vi "helper-unit-dose.vi"(6 "Auto Update Limit Record? (T)":bool=TRUE, 8 "error in":errorcluster, 9 "output":string, 10 "Unit Index":i32, 11 "Proc Name":string) -> (0 "error out":errorcluster, 1 "resulting string":string, 2 "Actual Dose in Seconds":i32)   [LabVIEW 2024]
uses:
  controls/enum-ntr-io-format.ctl
  globals/globals-engine.vi
panel:
  out "dose counter":dbl
  out "Daily Limit":dbl
  out "required dose":dbl
  out "ShouldDose":bool
  # "using unitIndex and output arguments this vi will check the daily limit to calculate the dose.\nreturn 0:  if limit is reached (meaning zero dose is no dose)\nretun X: where (0 < X <= doseTime) if limit isn't reached for today\nand keep a log of the process"
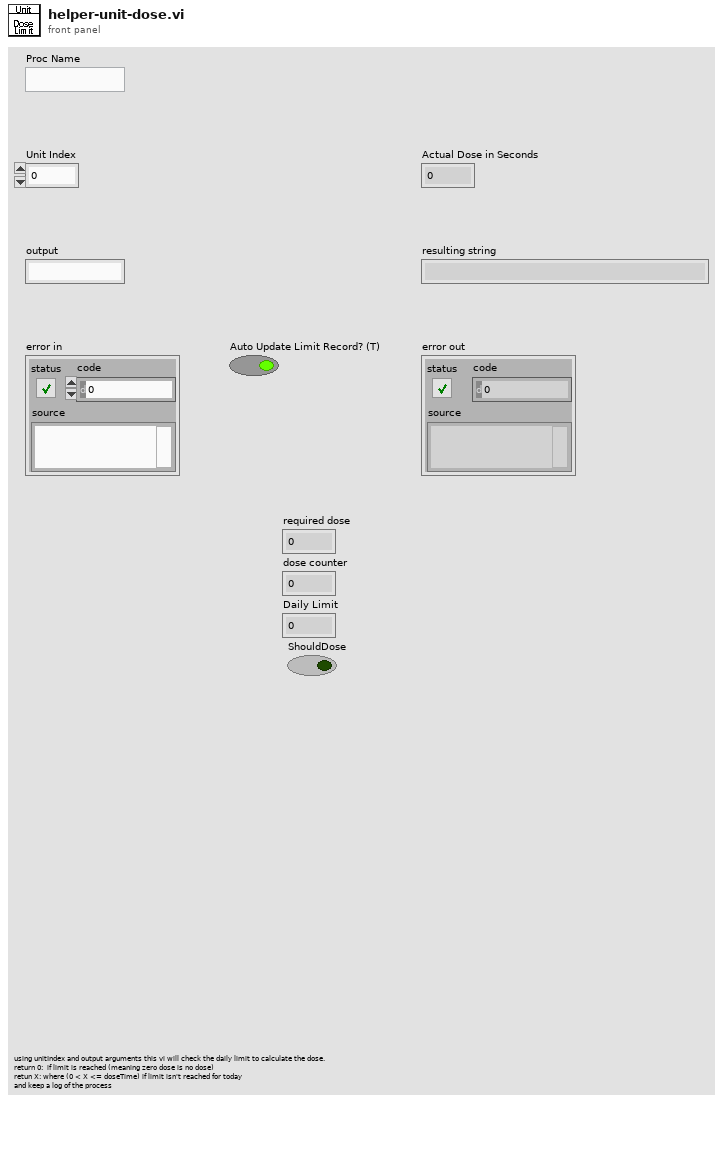
[diagram p1: front panel]
types:
  T1 = typedef "enum-ntr-io-format.ctl" = enum16{"UN_VLV%d", "UN_PMP%d", "UN_WL%d", "UN_PH", "UN_EC", "UN_ORP", "UN_WT", "UN_PH2", "UN_ALFA1", "UN_BETA1", "UN_ALFA2", "UN_BETA2", "UN_ACID", "UN_BASE", "UN_WATER", "UN_ORPMIX"}
  T2 = typedef "UiNutritionPanel.ctl" = cluster{"Main":cluster{"Enable":bool, "WashTimes":cluster{"In":dbl, "Out":dbl}, "DailyActivityHours":cluster{"Begin Time":T3, "End Time":T3}[]}, "Water Dosing":cluster{"Water Dose":dbl, "Water Limit":dbl}, "EC Ranges":cluster{"H Alarm":dbl, "L Alarm":dbl, "Low":dbl}, "EC Dosing":cluster{"ALFA1 Dose":dbl, "ALFA1 Limit":dbl, "BETA1 Dose":dbl, "BETA1 Limit":dbl, "ALFA2 Dose":dbl, "ALFA2 Limit":dbl, "BETA2 Dose":dbl, "BETA2 Limit":dbl}, "PH Ranges":cluster{"H Alarm":dbl, "L Alarm":dbl, "High":dbl, "Low":dbl}, "PH Dosing":cluster{"ACID Dose":dbl, "ACID Limit":dbl, "BASE Dose":dbl, "BASE Limit":dbl}, "ORP Ranges":cluster{"H Alarm":dbl, "L Alarm":dbl, "Low":dbl}, "ORP Dosing":cluster{"MIX Dose":dbl, "MIX Limit":dbl}}
  T3 = typedef "UiScheduleTimestamp.ctl" = timestamp
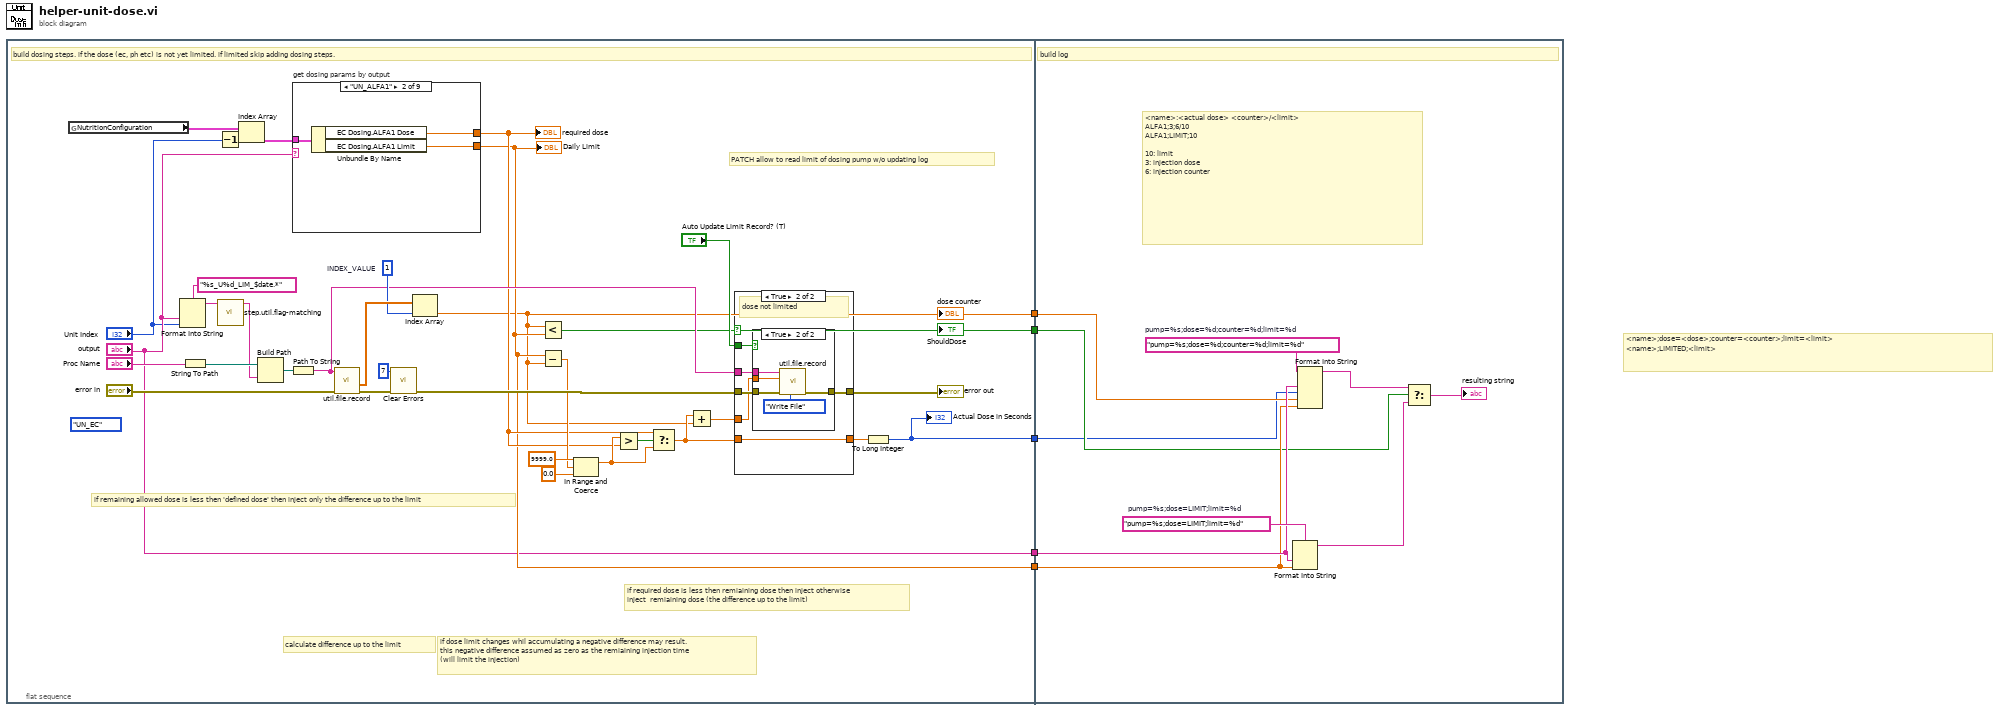
[diagram p0: block diagram]
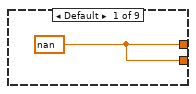
[diagram p2: hidden frame]
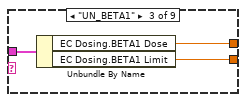
[diagram p3: hidden frame]
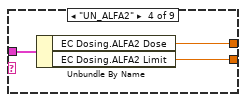
[diagram p4: hidden frame]
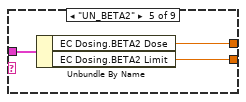
[diagram p5: hidden frame]
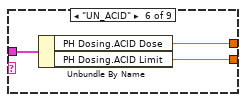
[diagram p6: hidden frame]
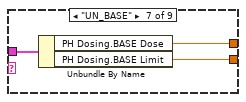
[diagram p7: hidden frame]
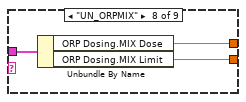
[diagram p8: hidden frame]
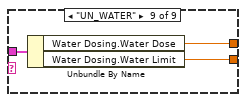
[diagram p9: hidden frame]
diagram:
  # "<name>;dose=<dose>;counter=<counter>;limit=<limit>\n<name>;LIMITED;<limit>"
  n1 = flat-sequence {
    tunnel: ["output"] -> w5
    tunnel: [w11] -> w4
    tunnel: [w10] -> w3
    tunnel: [w9] -> w2
    tunnel: [w8] -> w1
    tunnel: w5 -> [w81]
    tunnel: w4 -> [w80]
    tunnel: w3 -> [w79]
    tunnel: w2 -> [w78]
    tunnel: w1 -> [w77]
    frame #0 {
      (unwired) enum-ntr-io-format."UN_EC"
      w35 = 1  # INDEX_VALUE
      # "PATCH allow to read limit of dosing pump w/o updating log"
      # "if required dose is less then remiaining dose then inject otherwise\ninject  remiaining dose (the difference up to the limit)"
      # "if dose limit changes whil accumulating a negative difference may result.\nthis negative difference assumed as zero as the remiaining injection time \n(will limit the injection)"
      # "calculate difference up to the limit"
      # "if remaining allowed dose is less then 'defined dose' then inject only the difference up to the limit"
      # "build dosing steps. if the dose (ec, ph etc) is not yet limited. if limited skip adding dosing steps."
      n2 = global read "globals-engine.vi" "NutritionConfiguration"() -> (w12:T2[])
      n3 = Format Into String(format string="%s_U%d_LIM_$date.*", "output", "Unit Index") -> (resulting string=w25:string)  [unwired: 2 in, 1 out]
      n4 = String To Path(string="Proc Name") -> (path=w29:path)
      n5 = Decrement(x="Unit Index") -> (x-1=w22:i32)
      n6 = call "step.util.flag-matching.vi"("$string in"=w25) -> ("formated string out"=w24:string)  [unwired: 10 in]
      n7 = Index Array(array=w12, index=w22) -> (element=w21:T2)
      n8 = Build Path(base path=w29, name or relative path=w24) -> (appended path=w37:path)
      n9 = Path To String(path=w37) -> (string=w23:string)
      n10 = case "get dosing params by output" shown="\"UN_ALFA1\"" "output" {
        tunnel: w21 -> [_ w42 w45 w48 w51 w54 w57 w60 w63]
        tunnel: [w39 w41 w44 w47 w50 w53 w56 w59 w62] -> w15
        tunnel: [w39 w40 w43 w46 w49 w52 w55 w58 w61] -> w11
        frame Default {
          w39 = nan ("BETA2 Dose")
        }
        frame "UN_ALFA1" {
          n11 = Unbundle By Name(w42) -> ("EC Dosing.ALFA1 Dose"=w41:dbl, "EC Dosing.ALFA1 Limit"=w40:dbl)
        }
        frame "UN_BETA1" {
          n12 = Unbundle By Name(w45) -> ("EC Dosing.BETA1 Dose"=w44:dbl, "EC Dosing.BETA1 Limit"=w43:dbl)
        }
        frame "UN_ALFA2" {
          n13 = Unbundle By Name(w48) -> ("EC Dosing.ALFA2 Dose"=w47:dbl, "EC Dosing.ALFA2 Limit"=w46:dbl)
        }
        frame "UN_BETA2" {
          n14 = Unbundle By Name(w51) -> ("EC Dosing.BETA2 Dose"=w50:dbl, "EC Dosing.BETA2 Limit"=w49:dbl)
        }
        frame "UN_ACID" {
          n15 = Unbundle By Name(w54) -> ("PH Dosing.ACID Dose"=w53:dbl, "PH Dosing.ACID Limit"=w52:dbl)
        }
        frame "UN_BASE" {
          n16 = Unbundle By Name(w57) -> ("PH Dosing.BASE Dose"=w56:dbl, "PH Dosing.BASE Limit"=w55:dbl)
        }
        frame "UN_ORPMIX" {
          n17 = Unbundle By Name(w60) -> ("ORP Dosing.MIX Dose"=w59:dbl, "ORP Dosing.MIX Limit"=w58:dbl)
        }
        frame "UN_WATER" {
          n18 = Unbundle By Name(w63) -> ("Water Dosing.Water Dose"=w62:dbl, "Water Dosing.Water Limit"=w61:dbl)
        }
      }
      "required dose" <- w15
      "Daily Limit" <- w11
      n19 = call "util.file.record.vi"("error in"="error in", "path.* in"=w23) -> ("error out"=w34:errorcluster, "Last Record out"=w36:dbl[])  [unwired: 6 in, 2 out]
      n20 = call <vilib>:"Clear Errors.vi"("error in (no error)"=w34, "specific error code to clear (0: all)"=7) -> ("error out"=w32:errorcluster)  [unwired: 4 in, 1 out]
      n21 = Index Array(array=w36, index=w35) -> (element=w10:dbl)
      "dose counter" <- w10
      n22 = Less?(x=w10, y=w11) -> (x < y?=w9:bool)
      "ShouldDose" <- w9
      n23 = Subtract(x=w11, y=w10) -> (x-y=w16:dbl)
      n24 = In Range and Coerce(upper limit=9999.0, x=w16, lower limit=0.0) -> (coerced(x)=w18:dbl)  [unwired: 1 out]
      n25 = Greater?(x=w18, y=w15) -> (0:w38:bool)
      n26 = Select(t=w15, s=w38, f=w18) -> (s? t:f=w31:dbl)
      n27 = Add(x=w31, y=w10) -> (x+y=w30:dbl)
      n28 = case shown="True" w9 {
        tunnel: w32 -> [w64 w70]
        tunnel: w23 -> [_ w69]
        tunnel: w31 -> [_ w68]
        tunnel: [_ w68] -> w14
        tunnel: w30 -> [_ w67]
        tunnel: [w64 w66] -> w27
        tunnel: "Auto Update Limit Record? (T)" -> [_ w65]
        frame False {
          # "dose limited"
        }
        frame True {
          # "dose not limited"
          n29 = case shown="True" w65 {
            tunnel: w70 -> [w71 w75]
            tunnel: w69 -> [_ w74]
            tunnel: w67 -> [_ w73]
            tunnel: [w71 w72] -> w66
            frame False {
            }
            frame True {
              n30 = call "util.file.record.vi"("Operation(Read)"=enum16{"Read File", "Write File"}."Write File", "error in"=w75, "value"=w73, "path.* in"=w74) -> ("error out"=w72:errorcluster)  [unwired: 4 in, 3 out]
            }
          }
        }
      }
      "error out" <- w27
      n31 = To Long Integer(number=w14) -> (32bit integer=w8:i32)
      "Actual Dose in Seconds" <- w8
    }
    frame #1 {
      w83 = "pump=%s;dose=LIMIT;limit=%d"  # pump=%s;dose=LIMIT;limit=%d
      w84 = "pump=%s;dose=%d;counter=%d;limit=%d"  # pump=%s;dose=%d;counter=%d;limit=%d
      # "<name>:<actual dose> <counter>/<limit>\nALFA1;3;6/10\nALFA1;LIMIT;10\n\n10: limit\n3: injection dose\n6: injection counter"
      # "build log"
      n32 = Format Into String(format string=w83, w81, w80) -> (resulting string=w82:string)  [unwired: 2 in, 1 out]
      n33 = Format Into String(format string=w84, w81, w77, w79, w80) -> (resulting string=w85:string)  [unwired: 2 in, 1 out]
      n34 = Select(t=w85, s=w78, f=w82) -> (s? t:f=→"resulting string":string)
    }
  }
